vi "Write DMA.vi"(8 "error in (no error)":errorcluster, 10 "Refs":T1={"Data Type"=enum."I32", "DMA_SGL"=refnum, "DMA_U64"=refnum, "DMA_I64"=refnum, "DMA_FXP+/-32.8"=refnum, "DMA_FXP+/-64.32"=refnum, "DMA_U32"=refnum, "DMA_U16"=refnum, "DMA_U8"=refnum, "DMA_I32"=refnum, "DMA_I16"=refnum, "DMA_I8"=refnum, "DMA_FXP+/-32.16"=refnum} {"Data Type" format="%.0x"}, 11 "Waveform Refs":refnum<class "Single Waveform Read (DBL).lvclass">[](array[class])) -> (0 "error out":errorcluster, 1 "Empty Elements Remaining":u32, 2 "Refs out":T1={"Data Type"=enum."I32", "DMA_SGL"=refnum, "DMA_U64"=refnum, "DMA_I64"=refnum, "DMA_FXP+/-32.8"=refnum, "DMA_FXP+/-64.32"=refnum, "DMA_U32"=refnum, "DMA_U16"=refnum, "DMA_U8"=refnum, "DMA_I32"=refnum, "DMA_I16"=refnum, "DMA_I8"=refnum, "DMA_FXP+/-32.16"=refnum} {"Data Type" format="%.0x"}, 3 "Waveform Refs":refnum<class "Single Waveform Read (DBL).lvclass">[](array[class]))   [LabVIEW 2018, in "FPGA Addon Engine.lvlib"]
uses:
  FPGA Addon Engine.lvlib
  <vilib>/NI VeriStand/Custom Device Waveform API/NI_VS Custom Device Waveform API.lvlib
  <vilib>/rvi/interface/nirviMethod/nirviMethod.xnode
  <vilib>/FPGAPlugInAG/Dynamic/niLvFpga_WriteFifo_Dynamic.vi
  <vilib>/rvi/errors/niLvFpgaMergeErrorWithErrorCode.vi
  <vilib>/NI VeriStand/Custom Device Waveform API/Single Waveform Read (DBL)/NI VeriStand - Read Single Waveform (DBL).vi
  <vilib>/NI VeriStand/Custom Device Waveform API/Single Waveform Read (DBL)/Single Waveform Read (DBL).lvclass
  Types/DMA Output Refs.ctl
  Addon Shared/Types/Data Type.ctl
  Addon Shared/FPGA Addon Shared.lvlib
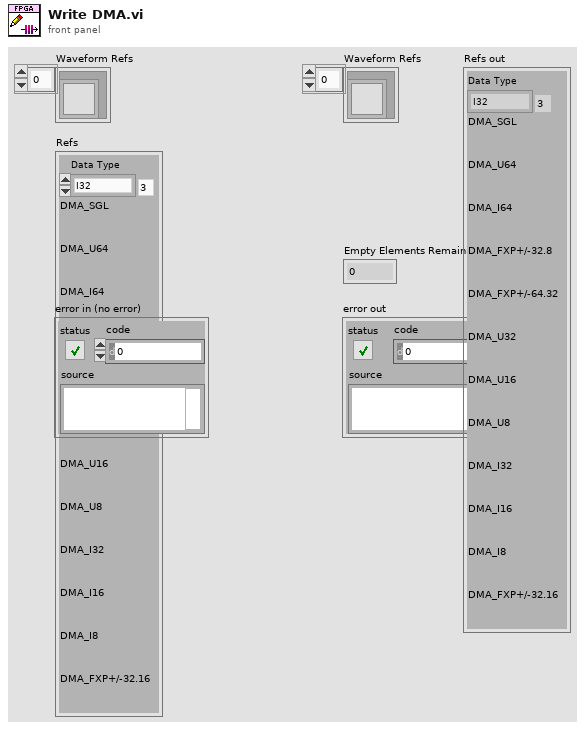
[diagram p1: front panel]
types:
  T1 = typedef "FPGA Addon Engine.lvlib/DMA Output Refs.ctl" = cluster{"Data Type":T2, "DMA_SGL":refnum<k20>, "DMA_U64":refnum<k20>, "DMA_I64":refnum<k20>, "DMA_FXP+/-32.8":refnum<k20>, "DMA_FXP+/-64.32":refnum<k20>, "DMA_U32":refnum<k20>, "DMA_U16":refnum<k20>, "DMA_U8":refnum<k20>, "DMA_I32":refnum<k20>, "DMA_I16":refnum<k20>, "DMA_I8":refnum<k20>, "DMA_FXP+/-32.16":refnum<k20>}
  T2 = typedef "FPGA Addon Shared.lvlib/Data Type.ctl" = enum8{"<Null>", "I8", "I16", "I32", "I64", "U8", "U16", "U32", "U64", "SGL", "Boolean", "Analog PWM In Settings", "Analog PWM In", "Digital PWM In Settings", "Digital PWM In", "Digital PWM Out", "Sine Out", "FXP+/-24.5", "FXP+/-16.5", "FXP+/-32.8", "FXP+/-64.32", "FXP+/-16.7", "FXP+/-20.5", "FXP+/-27.5", "FXP+/-32.16", "FXP+16.3", "FXP+18.3", "Digital Static In", "Digital Static Out", "Digital Static In Settings", "Digital WSS Out", "Quad Encoder Settings", "Quad Encoder In", "Group"}
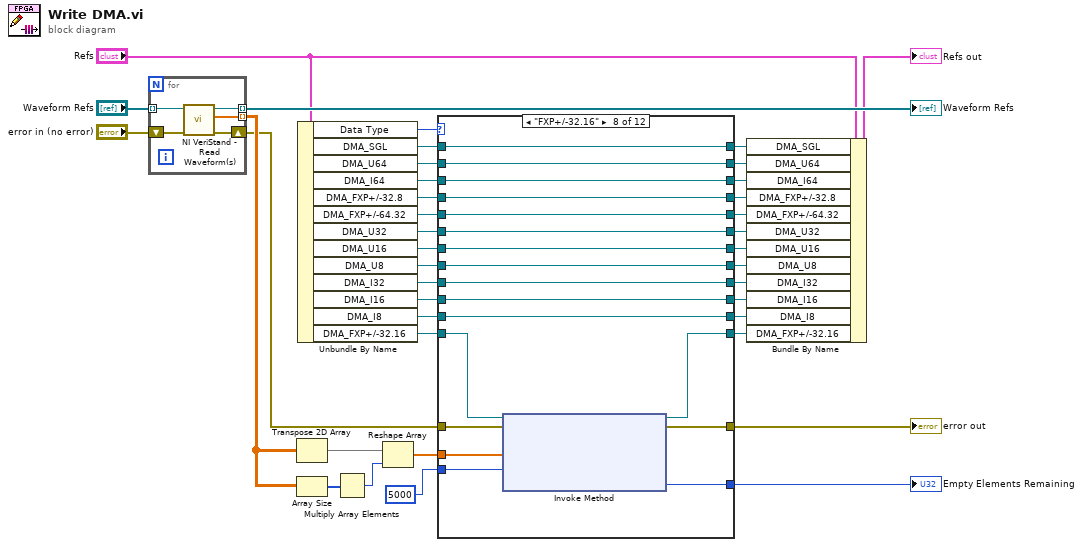
[diagram p0: block diagram]
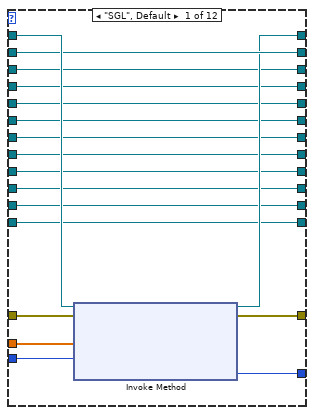
[diagram p2: hidden frame]
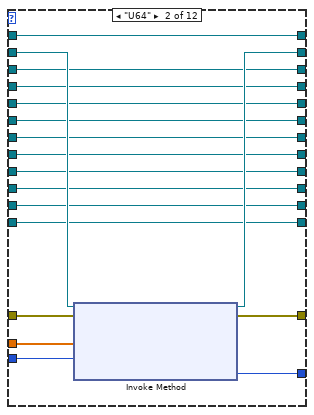
[diagram p3: hidden frame]
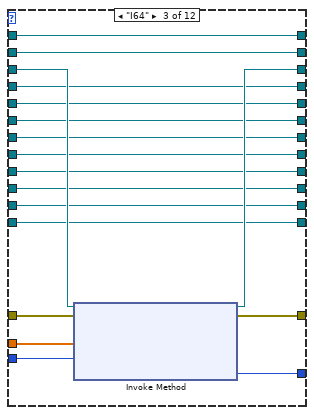
[diagram p4: hidden frame]
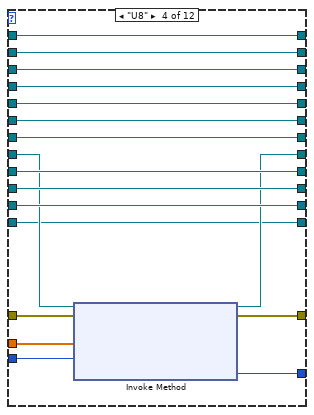
[diagram p5: hidden frame]
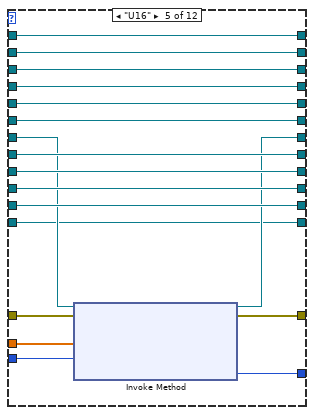
[diagram p6: hidden frame]
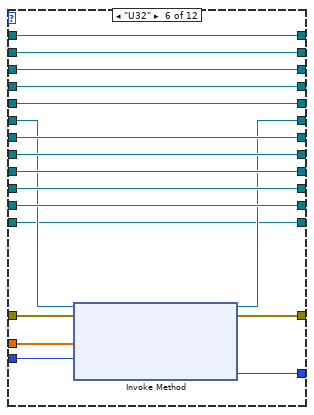
[diagram p7: hidden frame]
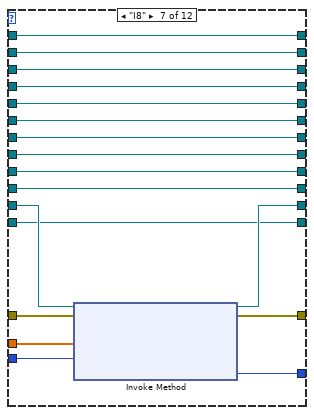
[diagram p8: hidden frame]
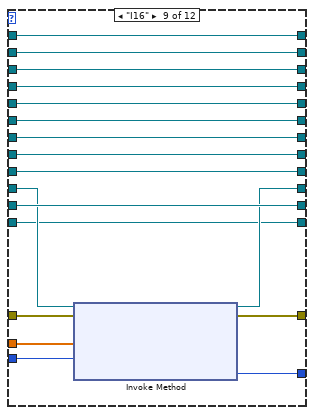
[diagram p9: hidden frame]
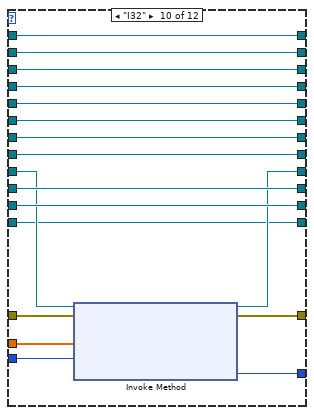
[diagram p10: hidden frame]
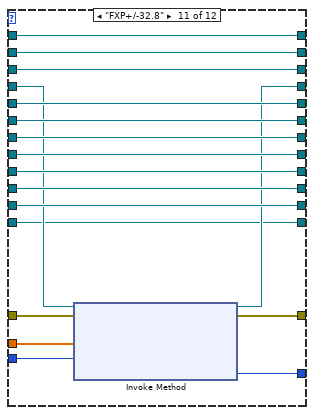
[diagram p11: hidden frame]
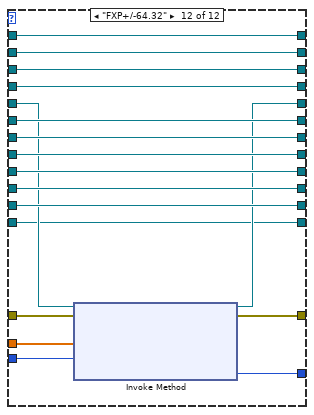
[diagram p12: hidden frame]
diagram:
  n1 = for {
    tunnel: [w44] -> w29 mode=indexing
    shift-right: [w43] -> w28
    shift-left: "error in (no error)" -> [w42]
    tunnel: "Waveform Refs" -> [w41] mode=indexing
    tunnel: [w40] -> w34 mode=indexing
    n2 = call-poly <vilib>:"NI VeriStand - Read Waveform(s).vi"("error in (no error)"=w42, "Single Waveform Read Session (DBL) in"=w41) -> ("error out"=w43:errorcluster, "Data"=w44:dbl[], "Single Waveform Read Session (DBL) out"=w40:refnum<class "Single Waveform Read (DBL).lvclass">)  [unwired: 5 in, 2 out]
  }
  "Waveform Refs" <- w34
  n3 = Transpose 2D Array(2D array=w29) -> (transposed array=w30:dbl[][])
  n4 = Array Size(array=w29) -> (size(s)=w32:i32[])
  n5 = Unbundle By Name("Refs") -> ("Data Type"=w27:T2, "DMA_SGL"=w26:refnum<k20>, "DMA_U64"=w25:refnum<k20>, "DMA_I64"=w20:refnum<k20>, "DMA_FXP+/-32.8"=w17:refnum<k20>, "DMA_FXP+/-64.32"=w15:refnum<k20>, "DMA_U32"=w13:refnum<k20>, "DMA_U16"=w11:refnum<k20>, "DMA_U8"=w9:refnum<k20>, "DMA_I32"=w7:refnum<k20>, "DMA_I16"=w5:refnum<k20>, "DMA_I8"=w3:refnum<k20>, "DMA_FXP+/-32.16"=w2:refnum<k20>)
  n6 = Multiply Array Elements(1:w32) -> (0:w31:i32)
  n7 = Reshape Array(w30, w31) -> (w36:dbl[])
  n8 = case shown="\"FXP+/-32.16\"" w27 {
    tunnel: [w62 w80 w98 w116 w134 w152 w170 w188 w206 w224 w242 w260] -> w39
    tunnel: [w61 w79 w97 w115 w133 w151 w169 w187 w205 w223 w241 w259] -> w38
    tunnel: 5000 ("Timeout (ms)") -> [w60 w78 w96 w114 w132 w150 w168 w186 w204 w222 w240 w258]
    tunnel: w36 -> [w59 w77 w95 w113 w131 w149 w167 w185 w203 w221 w239 w257]
    tunnel: w28 -> [w58 w76 w94 w112 w130 w148 w166 w184 w202 w220 w238 w256]
    tunnel: w26 -> [w57 w75 w93 w111 w129 w147 w165 w183 w201 w219 w237 w255]
    tunnel: [w56 w73 w90 w110 w128 w146 w164 w182 w200 w218 w236 w254] -> w23
    tunnel: w25 -> [w56 w74 w90 w110 w128 w146 w164 w182 w200 w218 w236 w254]
    tunnel: [w55 w75 w93 w111 w129 w147 w165 w183 w201 w219 w237 w255] -> w22
    tunnel: w20 -> [w54 w72 w92 w102 w120 w138 w156 w174 w192 w210 w228 w246]
    tunnel: [w54 w72 w91 w102 w120 w138 w156 w174 w192 w210 w228 w246] -> w19
    tunnel: [w46 w64 w89 w109 w127 w145 w163 w181 w199 w217 w226 w253] -> w18
    tunnel: w17 -> [w46 w64 w89 w109 w127 w145 w163 w181 w199 w217 w227 w253]
    tunnel: [w47 w65 w88 w108 w126 w144 w162 w180 w198 w216 w235 w244] -> w16
    tunnel: w15 -> [w47 w65 w88 w108 w126 w144 w162 w180 w198 w216 w235 w245]
    tunnel: [w48 w66 w87 w107 w125 w136 w161 w179 w197 w215 w234 w252] -> w14
    tunnel: w13 -> [w48 w66 w87 w107 w125 w137 w161 w179 w197 w215 w234 w252]
    tunnel: [w49 w67 w86 w106 w118 w143 w160 w178 w196 w214 w233 w251] -> w12
    tunnel: w11 -> [w49 w67 w86 w106 w119 w143 w160 w178 w196 w214 w233 w251]
    tunnel: [w50 w68 w85 w100 w124 w142 w159 w177 w195 w213 w232 w250] -> w10
    tunnel: w9 -> [w50 w68 w85 w101 w124 w142 w159 w177 w195 w213 w232 w250]
    tunnel: [w51 w69 w84 w105 w123 w141 w158 w176 w194 w208 w231 w249] -> w8
    tunnel: w7 -> [w51 w69 w84 w105 w123 w141 w158 w176 w194 w209 w231 w249]
    tunnel: [w52 w70 w83 w104 w122 w140 w157 w175 w190 w212 w230 w248] -> w6
    tunnel: w5 -> [w52 w70 w83 w104 w122 w140 w157 w175 w191 w212 w230 w248]
    tunnel: [w53 w71 w82 w103 w121 w139 w154 w171 w193 w211 w229 w247] -> w4
    tunnel: w3 -> [w53 w71 w82 w103 w121 w139 w155 w171 w193 w211 w229 w247]
    tunnel: w2 -> [w45 w63 w81 w99 w117 w135 w153 w173 w189 w207 w225 w243]
    tunnel: [w45 w63 w81 w99 w117 w135 w153 w172 w189 w207 w225 w243] -> w1
    frame "SGL", Default {
      n9 = xnode "Invoke Method"("FPGA VI Reference In"=w57, "error in"=w58, "Data"=w59, "Timeout (ms)"=w60) -> ("FPGA VI Reference Out"=w55:refnum<k20>, "error out"=w62:errorcluster, "Empty Elements Remaining"=w61:u32)
    }
    frame "U64" {
      n10 = xnode "Invoke Method"("FPGA VI Reference In"=w74, "error in"=w76, "Data"=w77, "Timeout (ms)"=w78) -> ("FPGA VI Reference Out"=w73:refnum<k20>, "error out"=w80:errorcluster, "Empty Elements Remaining"=w79:u32)
    }
    frame "I64" {
      n11 = xnode "Invoke Method"("FPGA VI Reference In"=w92, "error in"=w94, "Data"=w95, "Timeout (ms)"=w96) -> ("FPGA VI Reference Out"=w91:refnum<k20>, "error out"=w98:errorcluster, "Empty Elements Remaining"=w97:u32)
    }
    frame "U8" {
      n12 = xnode "Invoke Method"("FPGA VI Reference In"=w101, "error in"=w112, "Data"=w113, "Timeout (ms)"=w114) -> ("FPGA VI Reference Out"=w100:refnum<k20>, "error out"=w116:errorcluster, "Empty Elements Remaining"=w115:u32)
    }
    frame "U16" {
      n13 = xnode "Invoke Method"("FPGA VI Reference In"=w119, "error in"=w130, "Data"=w131, "Timeout (ms)"=w132) -> ("FPGA VI Reference Out"=w118:refnum<k20>, "error out"=w134:errorcluster, "Empty Elements Remaining"=w133:u32)
    }
    frame "U32" {
      n14 = xnode "Invoke Method"("FPGA VI Reference In"=w137, "error in"=w148, "Data"=w149, "Timeout (ms)"=w150) -> ("FPGA VI Reference Out"=w136:refnum<k20>, "error out"=w152:errorcluster, "Empty Elements Remaining"=w151:u32)
    }
    frame "I8" {
      n15 = xnode "Invoke Method"("FPGA VI Reference In"=w155, "error in"=w166, "Data"=w167, "Timeout (ms)"=w168) -> ("FPGA VI Reference Out"=w154:refnum<k20>, "error out"=w170:errorcluster, "Empty Elements Remaining"=w169:u32)
    }
    frame "FXP+/-32.16" {
      n16 = xnode "Invoke Method"("FPGA VI Reference In"=w173, "error in"=w184, "Data"=w185, "Timeout (ms)"=w186) -> ("FPGA VI Reference Out"=w172:refnum<k20>, "error out"=w188:errorcluster, "Empty Elements Remaining"=w187:u32)
    }
    frame "I16" {
      n17 = xnode "Invoke Method"("FPGA VI Reference In"=w191, "error in"=w202, "Data"=w203, "Timeout (ms)"=w204) -> ("FPGA VI Reference Out"=w190:refnum<k20>, "error out"=w206:errorcluster, "Empty Elements Remaining"=w205:u32)
    }
    frame "I32" {
      n18 = xnode "Invoke Method"("FPGA VI Reference In"=w209, "error in"=w220, "Data"=w221, "Timeout (ms)"=w222) -> ("FPGA VI Reference Out"=w208:refnum<k20>, "error out"=w224:errorcluster, "Empty Elements Remaining"=w223:u32)
    }
    frame "FXP+/-32.8" {
      n19 = xnode "Invoke Method"("FPGA VI Reference In"=w227, "error in"=w238, "Data"=w239, "Timeout (ms)"=w240) -> ("FPGA VI Reference Out"=w226:refnum<k20>, "error out"=w242:errorcluster, "Empty Elements Remaining"=w241:u32)
    }
    frame "FXP+/-64.32" {
      n20 = xnode "Invoke Method"("FPGA VI Reference In"=w245, "error in"=w256, "Data"=w257, "Timeout (ms)"=w258) -> ("FPGA VI Reference Out"=w244:refnum<k20>, "error out"=w260:errorcluster, "Empty Elements Remaining"=w259:u32)
    }
  }
  "error out" <- w39
  "Empty Elements Remaining" <- w38
  n21 = Bundle By Name(cluster="Refs", "DMA_SGL"=w22, "DMA_U64"=w23, "DMA_I64"=w19, "DMA_FXP+/-32.8"=w18, "DMA_FXP+/-64.32"=w16, "DMA_U32"=w14, "DMA_U16"=w12, "DMA_U8"=w10, "DMA_I32"=w8, "DMA_I16"=w6, "DMA_I8"=w4, "DMA_FXP+/-32.16"=w1) -> (→"Refs out":T1)
